vi "ZK蠕动泵1操作.vi"(7 "是否启用通讯通知":bool, 8 "error in (no error)":errorcluster, 10 "蠕动泵1操作":T2 items=["蠕动泵正转"=2, "蠕动泵反转"=3, "蠕动泵停止"=4], 11 "Slave ID":T1) -> (0 "error out":errorcluster)   [LabVIEW 2016, in "质控单元V2.lvlib"]
uses:
  <vilib>/Plasmionique/MB Master/MB_Master/MB_Master.lvclass
  <vilib>/Plasmionique/MB Master/MB Master.lvlib
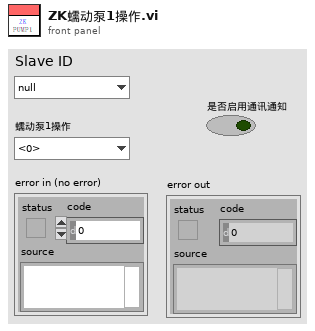
[diagram p1: front panel]
types:
  T1 = typedef "质控单元V2.lvlib/质控slave id.ctl" = enum16{"null", "氨氮", "总磷", "总氮", "CODMn", "CODCr"}
  T2 = typedef "质控单元V2.lvlib/质控蠕动泵操作.ctl" = u16
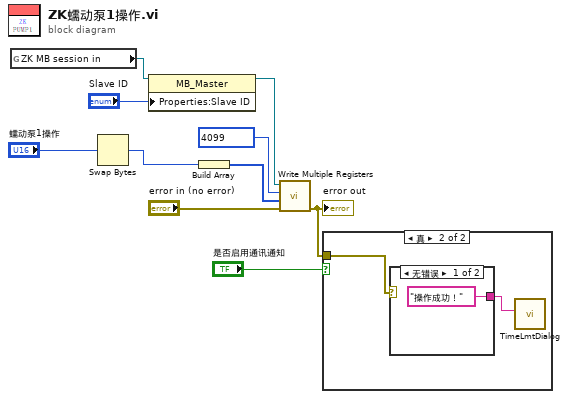
[diagram p0: block diagram]
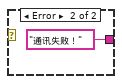
[diagram p3: hidden frame]
diagram:
  n1 = global read "ZK非断电保存全局变量.vi" "ZK MB session in"() -> (w9:refnum<class "MB_Master.lvclass">)
  n2 = Swap Bytes(anything="蠕动泵1操作") -> (byte swapped=w4:T2)
  n3 = property class="MB_Master"(reference=w9, "Properties:Slave ID"="Slave ID") -> (reference out=w6:refnum<class "MB_Master.lvclass">)  [unwired: 1 in, 1 out]
  n4 = Build Array(w4) -> (w3:T2[])
  n5 = call <vilib>:"Write Multiple Registers.vi"("error in (no error)"="error in (no error)", "values"=w3, "starting address"=u16 4099, "MB session in"=w6) -> ("error out"=w2:errorcluster)  [unwired: 6 in, 1 out]
  "error out" <- w2
  n6 = case shown="真" "是否启用通讯通知" {
    tunnel: w2 -> [_ w12]
    frame False {
    }
    frame True {
      n7 = case shown="无错误" w12 {
        tunnel: ["操作成功！" "通讯失败！"] -> w11
        frame No Error {
        }
        frame Error {
        }
      }
      n8 = call "TimeLmtDialog.vi"("Infoin"=w11) -> ()  [unwired: 11 in]
    }
  }
